vi "Boolean-Latch (SubVI).vi"(1 "Reset on First Call (T)":bool, 2 "Reset":bool, 3 "Trigger (Input)":bool) -> (0 "Latched? (Output)":bool)   [LabVIEW 2012]
panel:
  # "Boolean Latch (SubVI)"
  # "Blake Otting - Feb. 2007 - LabVIEW 8.2"
  # "This program takes a boolean (True or False) input and latches it \nON until the reset value is TRUE.\nThis is useful for making an intermittant signal constant."
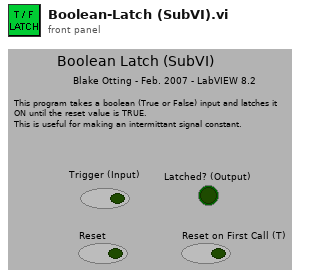
[diagram p1: front panel]
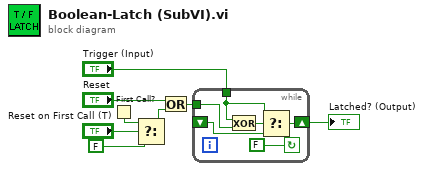
[diagram p0: block diagram]
diagram:
  n1 = First Call?() -> (First Call?: T/F=w5:bool)
  n2 = Select(t=w5, s="Reset on First Call (T)", f=FALSE) -> (s? t:f=w7:bool)
  n3 = Or(x="Reset", y=w7) -> (x .or. y?=w3:bool)
  n4 = while {
    tunnel: "Trigger (Input)" -> [w13]
    shift-right: [w11] -> w8
    shift-left: _ -> [w12]
    tunnel: w3 -> [w10]
    stop <- FALSE continue-if-true
    n5 = Exclusive Or(1:w10, 2:w13) -> (0:w14:bool)
    n6 = Select(t=w13, s=w14, f=w12) -> (s? t:f=w11:bool)
  }
  "Latched? (Output)" <- w8
